vi "InterruptControllerAbelTrap.vi"(4 "reference 4":refnum<vi>, 5 "FPGA VI Reference Out":refnum<k20>, 6 "reference 3":refnum<vi>, 7 "Bool Refnum":refnum<vi>, 9 "reference 2":refnum<vi>, 10 "reference":refnum<vi>, 11 "Boolean in":refnum<vi>) -> ()   [LabVIEW 2013]
uses:
  <vilib>/rvi/interface/common/niFpgaWaitOnOcc.vi
  <vilib>/Utility/error.llb/Error Cluster From Error Code.vi
  <vilib>/RVI Host/nirviSupport.llb/nirviErrorClusterFromErrorCode.vi
  <vilib>/rvi/errors/niLvFpgaAdjustHostInterfaceError.vi
  <vilib>/rvi/interface/nirviMethod/nirviMethod.xnode
  <vilib>/rvi/interface/nirviMethod/StockFPGA_InlinedMethodWaitForMultipleIRQ.vi
  <vilib>/FPGAPlugInAG/Dynamic/niLvFpga_WaitOnIrq_Dynamic.vi
  <vilib>/FPGAPlugInAG/Dynamic/niLvFpga_AcknowledgeIrq_Dynamic.vi
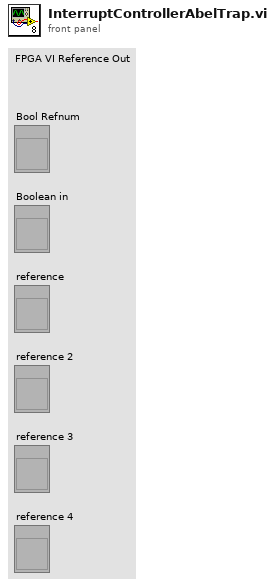
[diagram p1: front panel]
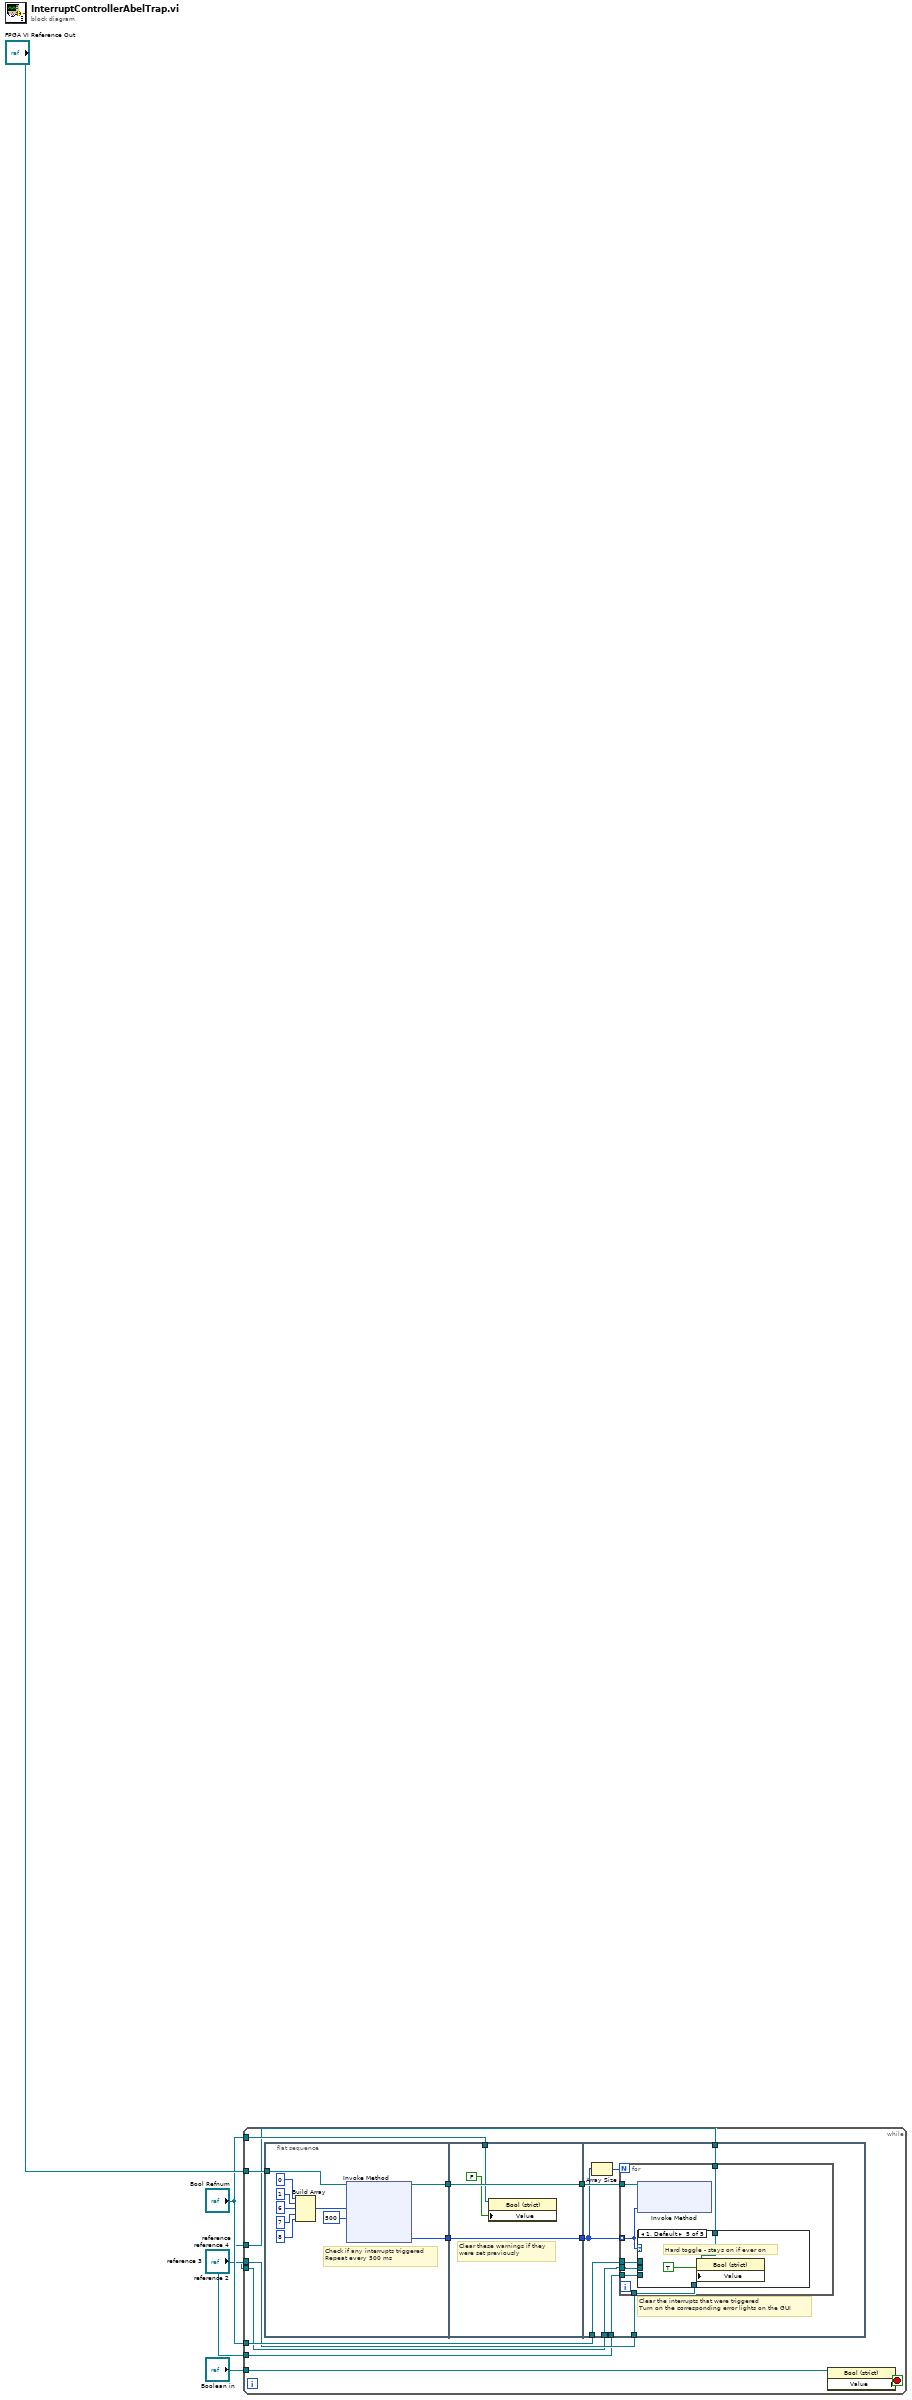
[diagram p0: block diagram]
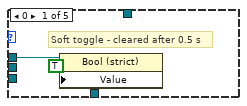
[diagram p2: hidden frame]
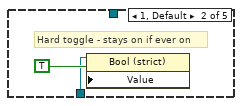
[diagram p3: hidden frame]
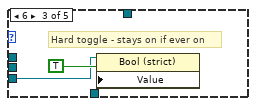
[diagram p4: hidden frame]
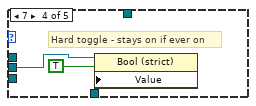
[diagram p5: hidden frame]
diagram:
  n1 = while {
    tunnel: "FPGA VI Reference Out" -> [w20]
    tunnel: "Bool Refnum" -> [w14]
    tunnel: "Bool Refnum" -> [w13]
    tunnel: "reference" -> [w12]
    tunnel: "reference 2" -> [w11]
    tunnel: "reference 3" -> [w10]
    tunnel: "reference 4" -> [w9]
    tunnel: "Boolean in" -> [w8]
    stop <- w15 stop-if-true
    n2 = flat-sequence {
      tunnel: w20 -> [w25]
      tunnel: [w22] -> w19
      tunnel: [w21] -> w17
      tunnel: w19 -> [w34]
      tunnel: [w34] -> w18
      tunnel: w17 -> [w33]
      tunnel: [w33] -> w16
      tunnel: w14 -> [w31]
      tunnel: w18 -> [w40]
      tunnel: w16 -> [w41]
      tunnel: w13 -> [w39]
      tunnel: w12 -> [w38]
      tunnel: w11 -> [w37]
      tunnel: w10 -> [w36]
      tunnel: w9 -> [w35]
      frame #0 {
        # "Check if any interrupts triggered\nRepeat every 500 ms"
        n3 = Build Array(0 ("element"), 1 ("element"), 6 ("element"), 7 ("element"), 8 ("element")) -> (w24:i32[])
        n4 = xnode "Invoke Method"("FPGA VI Reference In"=w25, "IRQ Number(s)"=w24, "Timeout (ms)"=500) -> ("FPGA VI Reference Out"=w21:refnum<k20>, "IRQ(s) Asserted"=w22:i32[])  [unwired: 1 in, 2 out]
      }
      frame #1 {
        # "Clear these warnings if they\nwere set previously"
        n5 = property on="Property Node" class="Bool (strict)"(reference=w31, "Value"=FALSE ("Mistimed")) -> ()  [unwired: 1 in, 2 out]
      }
      frame #2 {
        # "Clear the interrupts that were triggered\nTurn on the corresponding error lights on the GUI"
        n6 = Array Size(array=w40) -> (size(s)=w42:i32)
        n7 = for {
          N: w42 -> [_]
          tunnel: w41 -> [w49]
          tunnel: w40 -> [w48] mode=indexing
          tunnel: w39 -> [w47]
          tunnel: w38 -> [w46]
          tunnel: w37 -> [w45]
          tunnel: w36 -> [w44]
          tunnel: w35 -> [w43]
          n8 = xnode "Invoke Method"("FPGA VI Reference In"=w49, "IRQ Number(s)"=w48) -> ()  [unwired: 1 in, 2 out]
          n9 = case shown="1, Default" w48 {
            tunnel: w47 -> [w50 _ _ _ _]
            tunnel: w46 -> [_ w52 _ _ _]
            tunnel: w45 -> [_ _ w54 _ _]
            tunnel: w44 -> [_ _ _ w56 _]
            tunnel: w43 -> [_ _ _ _ w58]
            frame 0 {
              # "Soft toggle - cleared after 0.5 s"
              n10 = property class="Bool (strict)"(reference=w50, "Value"=TRUE ("Overflow")) -> ()  [unwired: 1 in, 2 out]
            }
            frame 1, Default {
              # "Hard toggle - stays on if ever on"
              n11 = property class="Bool (strict)"(reference=w52, "Value"=TRUE ("Incorrect Command")) -> ()  [unwired: 1 in, 2 out]
            }
            frame 6 {
              # "Hard toggle - stays on if ever on"
              n12 = property class="Bool (strict)"(reference=w54, "Value"=TRUE ("Mistimed")) -> ()  [unwired: 1 in, 2 out]
            }
            frame 7 {
              # "Hard toggle - stays on if ever on"
              n13 = property class="Bool (strict)"(reference=w56, "Value"=TRUE ("Mistimed")) -> ()  [unwired: 1 in, 2 out]
            }
            frame 8 {
              # "Hard toggle - stays on if ever on"
              n14 = property class="Bool (strict)"(reference=w58, "Value"=TRUE ("Mistimed")) -> ()  [unwired: 1 in, 2 out]
            }
          }
        }
      }
    }
    n15 = property class="Bool (strict)"(reference=w8) -> ("Value"=w15:bool)  [unwired: 1 in, 2 out]
  }
